vi "Read Timeout.vi"(8 "error in (no error)":errorcluster, 11 "Wait On Boolean Step Config in":refnum<class "Wait On Boolean Step Config.lvclass">) -> (0 "error out":errorcluster, 2 "Timeout":i32, 3 "Wait On Boolean Step Config out":refnum<class "Wait On Boolean Step Config.lvclass">)   [LabVIEW 2015, in "Wait On Boolean Step Config.lvclass"]
uses:
  Wait On Boolean Step Config.lvclass
  Wait On Boolean Step Config.lvclass/Wait On Boolean Step Config.ctl
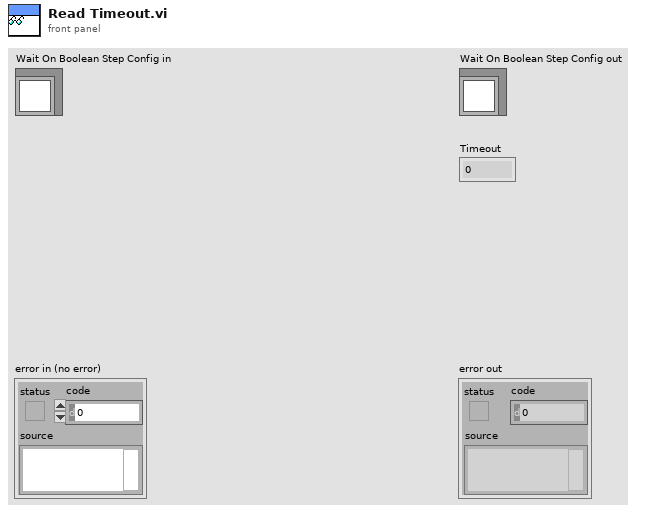
[diagram p1: front panel]
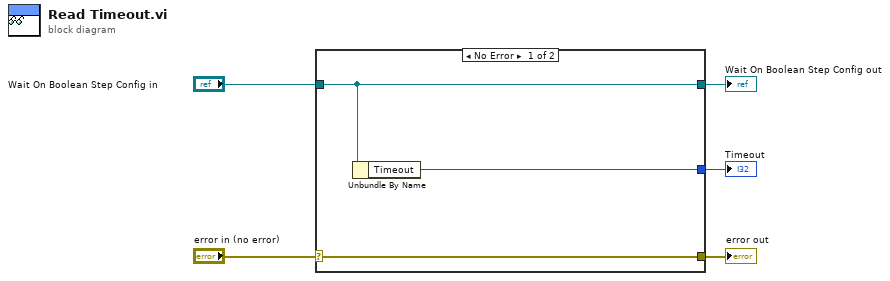
[diagram p0: block diagram]
diagram:
  n1 = case shown="No Error" "error in (no error)" {
    selector: "error in (no error)" -> [w8 w9]
    tunnel: [w8 w9] -> w4
    tunnel: [w7 w10] -> w2
    tunnel: "Wait On Boolean Step Config in" -> [w7 w10]
    tunnel: [w6 _] -> w1
    frame No Error {
      n2 = Unbundle By Name(w7) -> ("Timeout"=w6:i32)
    }
    frame Error {
    }
  }
  "error out" <- w4
  "Wait On Boolean Step Config out" <- w2
  "Timeout" <- w1
